vi "Write Debug Text String.vi"(10 "text":string) -> ()   [LabVIEW 2020, in "Regatron G5 Custom Device Engine.lvlib"]
uses:
  Regatron G5 Custom Device Engine.lvlib
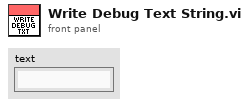
[diagram p1: front panel]
types:
  T1 = enum16{"open", "replace", "create", "open or create", "replace or create", "replace or create with confirmation"}
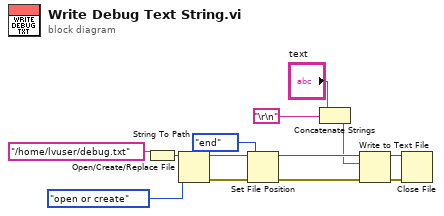
[diagram p0: block diagram]
diagram:
  n1 = String To Path(string="/home/lvuser/debug.txt") -> (path=w6:path)
  n2 = Open/Create/Replace File(file path (use dialog)=w6, operation (0:open)=T1."open or create") -> (refnum out=w13:refnum<file>, error out=w12:errorcluster)  [unwired: 4 in, 1 out]
  n3 = Set File Position(refnum=w13, from (0:start)=enum16{"start", "end", "current"}."end", error in=w12) -> (refnum out=w11:refnum<file>, error out=w10:errorcluster)  [unwired: 1 in]
  n4 = Concatenate Strings("text", "\r\n") -> (w2:string)
  n5 = Write to Text File(file (use dialog)=w11, text=w2, error in=w10) -> (refnum out=w9:refnum<file>, error out=w8:errorcluster)  [unwired: 1 in, 1 out]
  n6 = Close File(refnum=w9, error in=w8) -> ()  [unwired: 2 out]
